vi "Test ZMQ Context Manager.vi"() -> ()   [LabVIEW 2019, in "RemoteControl.ZMQ.lvlib" / "RemoteControl.ZMQ.lvclass"]
uses:
  RemoteControl.ZMQ.lvclass
  RemoteControl.ZMQ.lvclass/RemoteControl.ZMQ.ctl
  <userlib>/_OpenG.lib/time/time.llb/openg_time.lvlib
  ZMQ.ContextManager/ZMQ.ContextManager.lvlib
panel:
  out "error out":errorcluster
  # "Open block diagram and open ZMQ.ContextManager.\nRun Me and watch the counter:\n0: Force cleanup context DVR\n0 - 1 - 0: create and release context (without socket)\n0 - 1: create server socket (creates a context)\n1 - 2: create client socket\n2 - 3: create 2nd client socket\n3 - 2: close client socket\n2 - 1: close client socket\n1 - 0: close server socket"
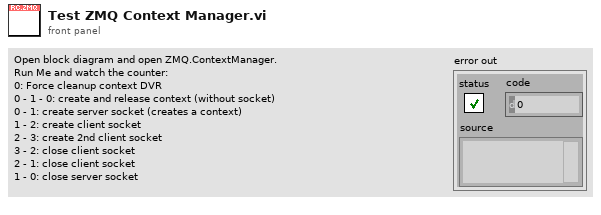
[diagram p1: front panel]
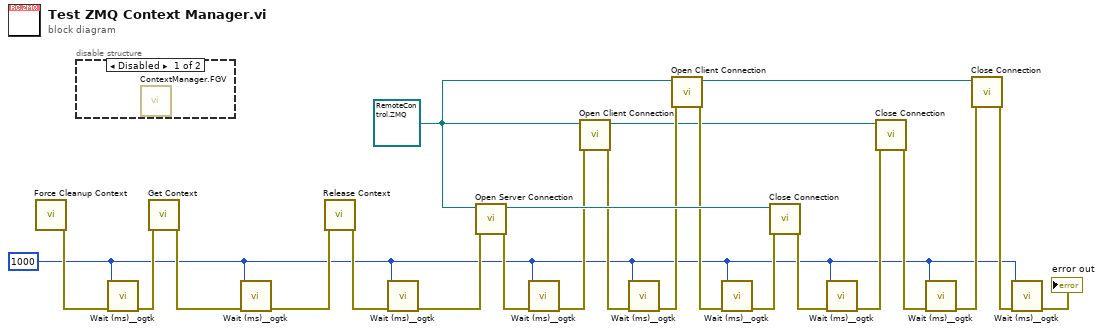
[diagram p0: block diagram]
diagram:
  w1 = u32 1000 ("milliseconds to wait")
  w14 = refnum<class "RemoteControl.ZMQ.lvclass"> refnum ("RemoteControl.ZMQ.lvlib:RemoteControl.ZMQ.lvclass")
  n1 = call "Force Cleanup Context.vi"() -> ("error out"=w4:errorcluster)  [unwired: 10 in, 1 out]
  n2 = disable-structure shown="Disabled" {
    frame Disabled {
      n3 = call "ContextManager.FGV.vi"() -> ()  [unwired: 10 in, 2 out]
    }
    frame Enabled {
    }
  }
  n4 = call <userlib>:"Wait (ms)__ogtk.vi"("error in (no error)"=w4, "milliseconds to wait"=w1) -> ("error out"=w3:errorcluster)  [unwired: 8 in, 1 out]
  n5 = call "Get Context.vi"("error in"=w3) -> ("error out"=w2:errorcluster)  [unwired: 9 in, 1 out]
  n6 = call <userlib>:"Wait (ms)__ogtk.vi"("error in (no error)"=w2, "milliseconds to wait"=w1) -> ("error out"=w21:errorcluster)  [unwired: 8 in, 1 out]
  n7 = call "Release Context.vi"("error in"=w21) -> ("error out"=w20:errorcluster)  [unwired: 9 in, 1 out]
  n8 = call <userlib>:"Wait (ms)__ogtk.vi"("error in (no error)"=w20, "milliseconds to wait"=w1) -> ("error out"=w19:errorcluster)  [unwired: 8 in, 1 out]
  n9 = call-dynamic "Open Server Connection.vi"("error in (no error)"=w19, "RemoteControl.ZMQ in"=w14) -> ("error out"=w18:errorcluster, "RemoteControl.ZMQ out"=w23:refnum<class "RemoteControl.ZMQ.lvclass">)  [unwired: 8 in]
  n10 = call <userlib>:"Wait (ms)__ogtk.vi"("error in (no error)"=w18, "milliseconds to wait"=w1) -> ("error out"=w17:errorcluster)  [unwired: 8 in, 1 out]
  n11 = call-dynamic "Open Client Connection.vi"("error in (no error)"=w17, "RemoteControl.ZMQ in"=w14) -> ("error out"=w13:errorcluster, "RemoteControl.ZMQ out"=w9:refnum<class "RemoteControl.ZMQ.lvclass">)  [unwired: 8 in]
  n12 = call <userlib>:"Wait (ms)__ogtk.vi"("error in (no error)"=w13, "milliseconds to wait"=w1) -> ("error out"=w12:errorcluster)  [unwired: 8 in, 1 out]
  n13 = call-dynamic "Open Client Connection.vi"("error in (no error)"=w12, "RemoteControl.ZMQ in"=w14) -> ("error out"=w11:errorcluster, "RemoteControl.ZMQ out"=w10:refnum<class "RemoteControl.ZMQ.lvclass">)  [unwired: 8 in]
  n14 = call <userlib>:"Wait (ms)__ogtk.vi"("error in (no error)"=w11, "milliseconds to wait"=w1) -> ("error out"=w22:errorcluster)  [unwired: 8 in, 1 out]
  n15 = call-dynamic "Close Connection.vi"("error in (no error)"=w22, "RemoteControl.ZMQ in"=w23) -> ("error out"=w16:errorcluster)  [unwired: 8 in, 1 out]
  n16 = call <userlib>:"Wait (ms)__ogtk.vi"("error in (no error)"=w16, "milliseconds to wait"=w1) -> ("error out"=w15:errorcluster)  [unwired: 8 in, 1 out]
  n17 = call-dynamic "Close Connection.vi"("error in (no error)"=w15, "RemoteControl.ZMQ in"=w9) -> ("error out"=w8:errorcluster)  [unwired: 8 in, 1 out]
  n18 = call <userlib>:"Wait (ms)__ogtk.vi"("error in (no error)"=w8, "milliseconds to wait"=w1) -> ("error out"=w7:errorcluster)  [unwired: 8 in, 1 out]
  n19 = call-dynamic "Close Connection.vi"("error in (no error)"=w7, "RemoteControl.ZMQ in"=w10) -> ("error out"=w6:errorcluster)  [unwired: 8 in, 1 out]
  n20 = call <userlib>:"Wait (ms)__ogtk.vi"("error in (no error)"=w6, "milliseconds to wait"=w1) -> ("error out"=→"error out":errorcluster)  [unwired: 8 in, 1 out]
